vi "Get DIO Lines.vi"(8 "error in (no error)":errorcluster, 10 "path to XML document":path, 11 "RIO Target in":refnum<class "RIO Target.lvclass">) -> (0 "error out":errorcluster, 2 "DIO Lines":string[](array[string]), 3 "RIO Target out":refnum<class "RIO Target.lvclass">)   [LabVIEW 2014, in "RIO Target.lvclass"]
uses:
  RIO Target.lvclass
  <vilib>/xml/Load XML File.vi
  <vilib>/xml/Close Reference(Node).vi
  <vilib>/xml/Close Reference(NNMap).vi
  <vilib>/xml/Close Reference(NdList).vi
  <vilib>/xml/NI_XML.lvlib
  <resource>/objmgr/DOMUserDefRef.rc
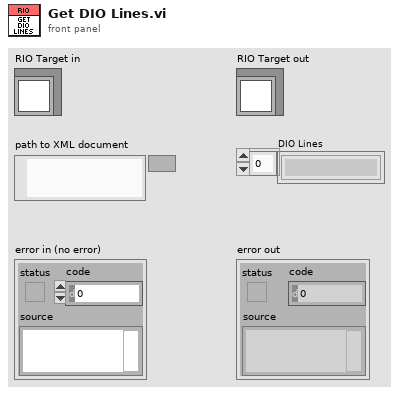
[diagram p1: front panel]
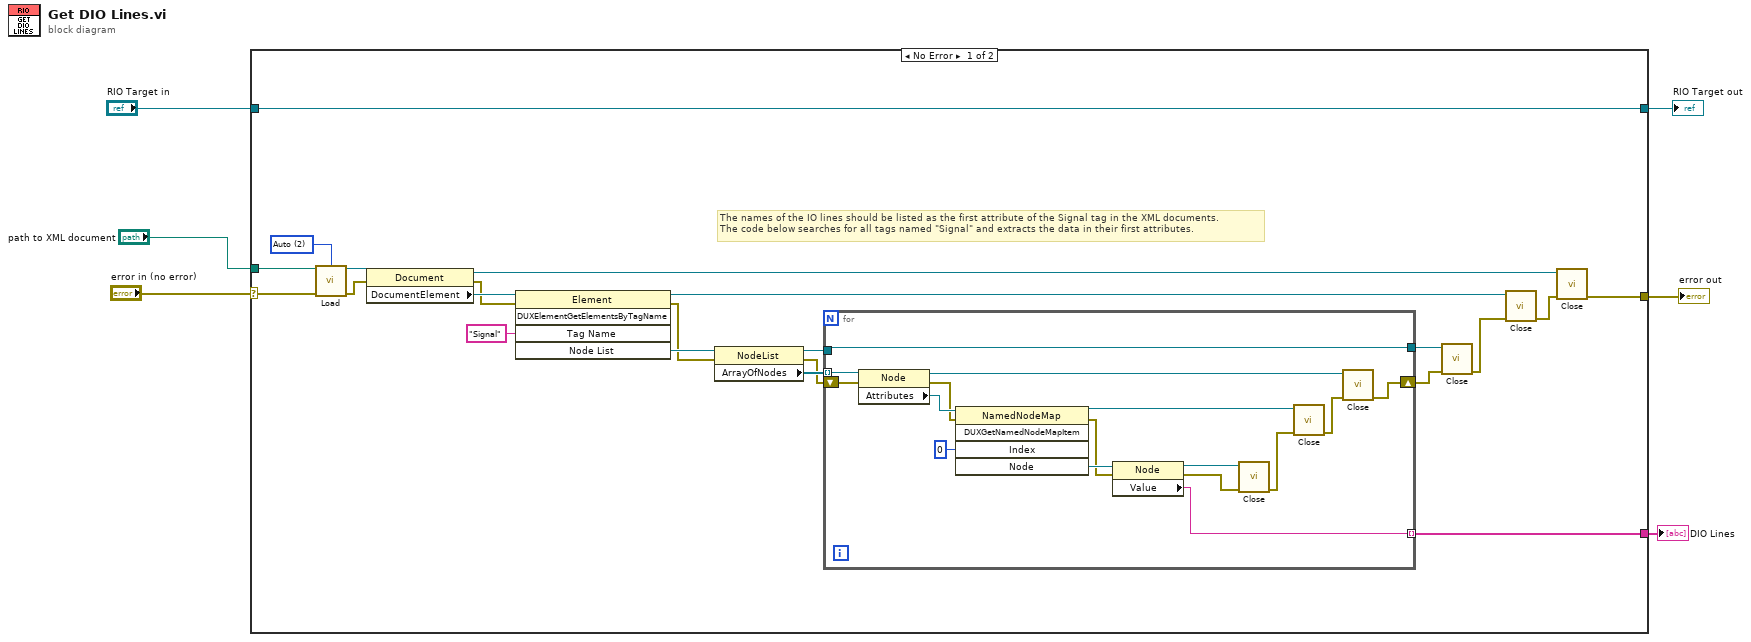
[diagram p0: block diagram]
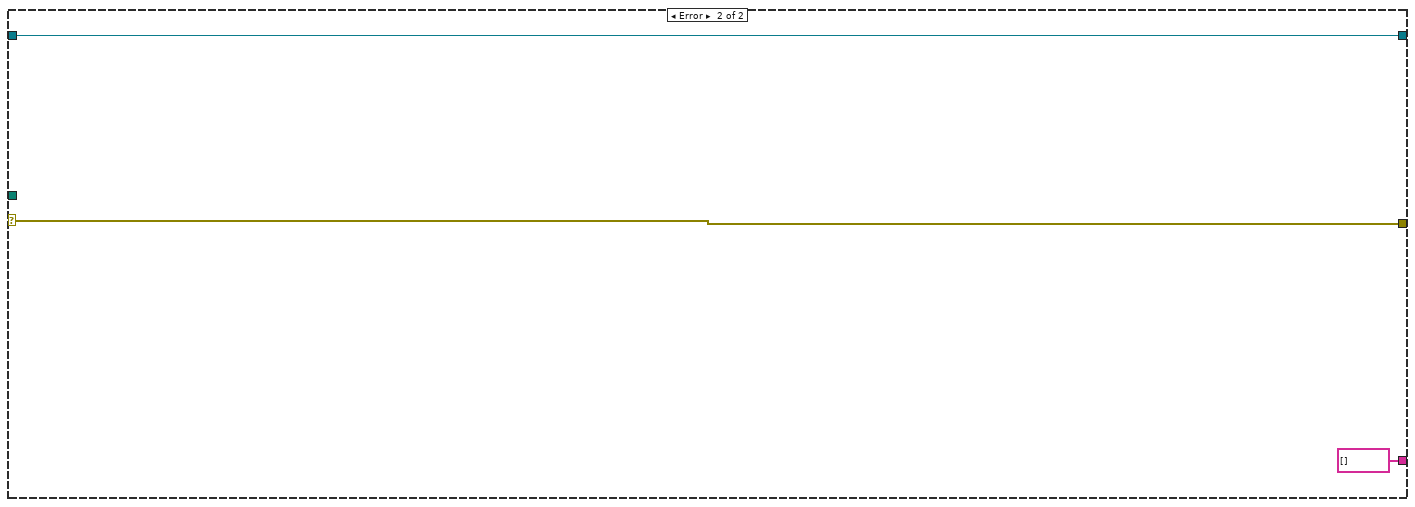
[diagram p2: hidden frame]
diagram:
  n1 = case shown="No Error" "error in (no error)" {
    selector: "error in (no error)" -> [w10 w47]
    tunnel: [w8 w47] -> w2
    tunnel: [w28 w46] -> w4
    tunnel: "RIO Target in" -> [w28 w46]
    tunnel: "path to XML document" -> [w9 _]
    tunnel: [w7 string[] []] -> w1
    frame No Error {
      w27 = 2 items=["Never", "Always", "Auto"] ("validate on load (Auto)")
      # "The names of the IO lines should be listed as the first attribute of the Signal tag in the XML documents. \nThe code below searches for all tags named \"Signal\" and extracts the data in their first attributes."
      n2 = call-poly <vilib>:"Load.vi"("path to XML document"=w9, "validate on load (Auto)"=w27, "error in (no error)"=w10) -> ("DOM document out"=w26:refnum<k20>, "error out"=w23:errorcluster)  [unwired: 10 in, 1 out]
      n3 = property class="Document"(reference=w26, error in=w23) -> (reference out=w17:refnum<k20>, error out=w22:errorcluster, "DocumentElement"=w25:refnum<k20>)
      n4 = invoke class="Element" method="DUXElementGetElementsByTagName"(reference=w25, error in=w22, "Tag Name"="Signal") -> (reference out=w18:refnum<k20>, error out=w16:errorcluster, "Node List"=w21:refnum<k20>)  [unwired: 2 in, 2 out]
      n5 = property class="NodeList"(reference=w21, error in=w16) -> (reference out=w15:refnum<k20>, error out=w14:errorcluster, "ArrayOfNodes"=w20:refnum<k20>[])
      n6 = for {
        tunnel: w20 -> [w31] mode=indexing
        tunnel: w15 -> [w32]
        shift-right: [w29] -> w13
        shift-left: w14 -> [w30]
        tunnel: [w41] -> w7 mode=indexing
        tunnel: [w32] -> w11
        n7 = property class="Node"(reference=w31, error in=w30) -> (reference out=w37:refnum<k20>, error out=w43:errorcluster, "Attributes"=w44:refnum<k20>)
        n8 = invoke class="NamedNodeMap" method="DUXGetNamedNodeMapItem"(reference=w44, error in=w43, "Index"=0) -> (reference out=w36:refnum<k20>, error out=w35:errorcluster, "Node"=w42:refnum<k20>)  [unwired: 2 in, 2 out]
        n9 = property class="Node"(reference=w42, error in=w35) -> (reference out=w34:refnum<k20>, error out=w40:errorcluster, "Value"=w41:string)
        n10 = call-poly <vilib>:"Close.vi"("error in (no error)"=w40, "node"=w34) -> ("error out"=w39:errorcluster)  [unwired: 7 out]
        n11 = call-poly <vilib>:"Close.vi"("error in (no error)"=w39, "named node map"=w36) -> ("error out"=w38:errorcluster)  [unwired: 7 out]
        n12 = call-poly <vilib>:"Close.vi"("error in (no error)"=w38, "node"=w37) -> ("error out"=w29:errorcluster)  [unwired: 7 out]
      }
      n13 = call-poly <vilib>:"Close.vi"("error in (no error)"=w13, "node list"=w11) -> ("error out"=w12:errorcluster)  [unwired: 7 out]
      n14 = call-poly <vilib>:"Close.vi"("error in (no error)"=w12, "node"=w18) -> ("error out"=w19:errorcluster)  [unwired: 7 out]
      n15 = call-poly <vilib>:"Close.vi"("error in (no error)"=w19, "node"=w17) -> ("error out"=w8:errorcluster)  [unwired: 7 out]
    }
    frame Error {
    }
  }
  "error out" <- w2
  "RIO Target out" <- w4
  "DIO Lines" <- w1
